vi "Select Searching Method.vi"(8 "error in (no error)":errorcluster) -> (0 "error out":errorcluster, 1 "To Date Field":string, 2 "From Date Field":string, 3 "Selection Type":string)   [LabVIEW 2017]
panel:
  out "Description":string
  in  "Search Type":string(combo)="Date&Time"
  in  "Select":bool
  in  "OK":bool
  # "o selecting this method you can search the"
  # "Select The Searching Method"
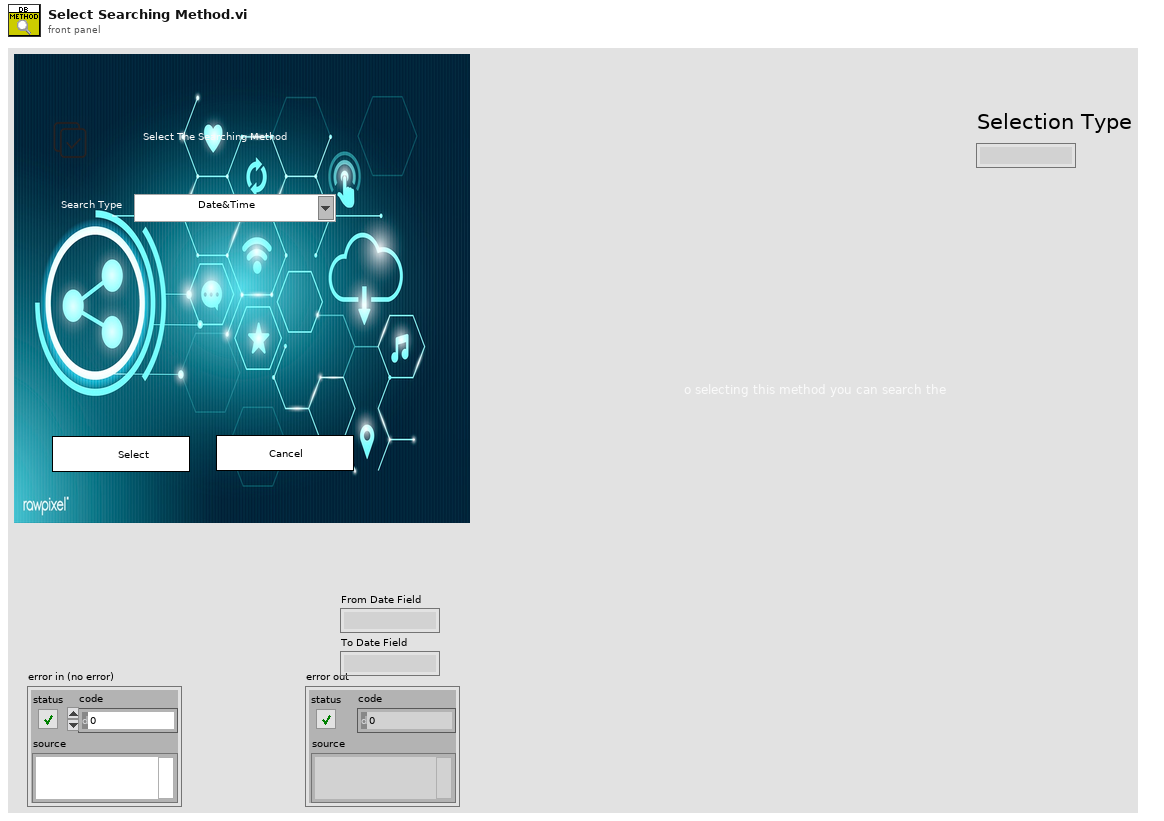
[diagram p1: front panel]
types:
  T1 = cluster{"Search Type":string, "Old Selection Type":string, "Description":string}
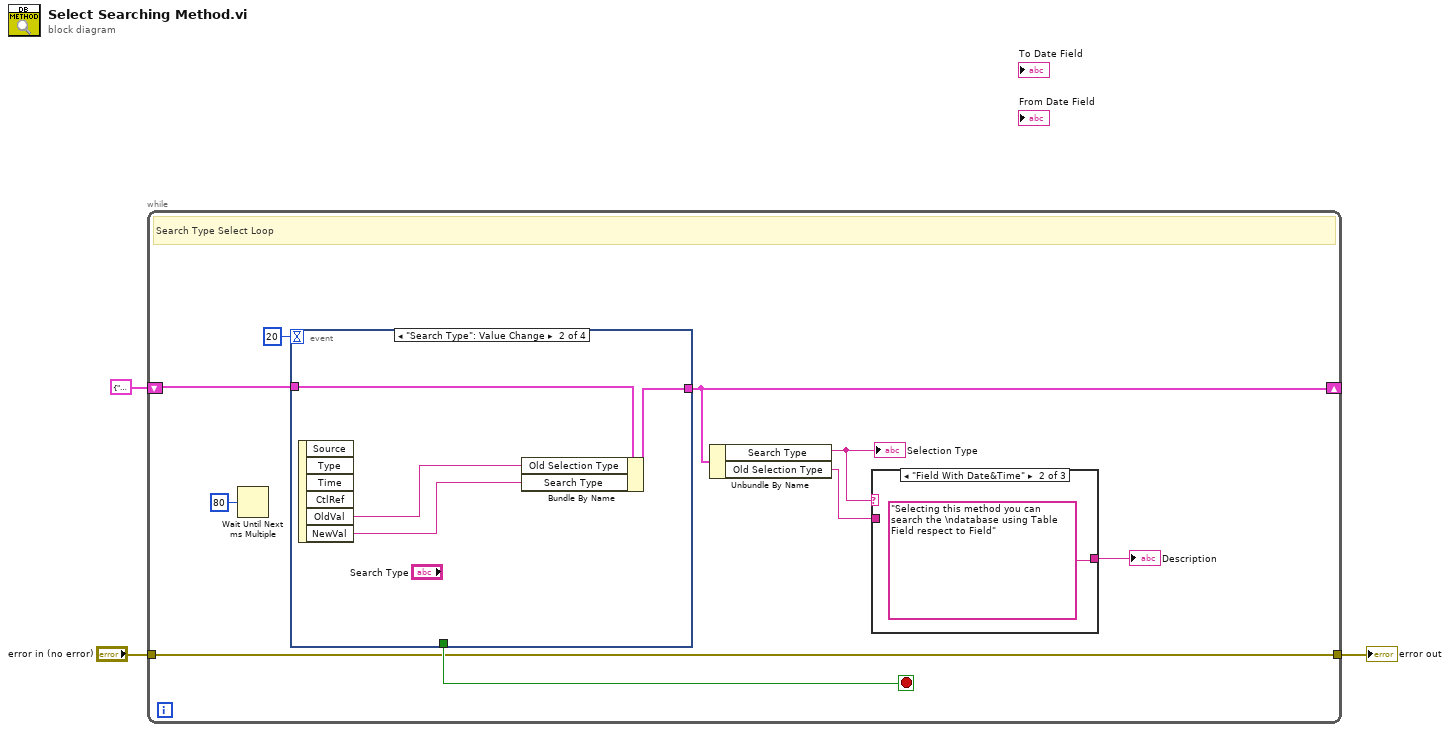
[diagram p0: block diagram]
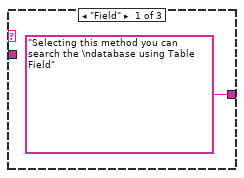
[diagram p2: hidden frame]
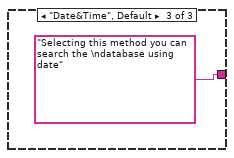
[diagram p3: hidden frame]
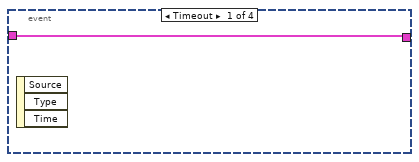
[diagram p4: hidden frame]
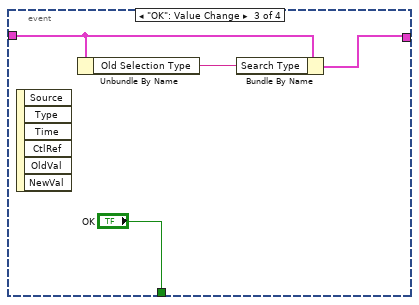
[diagram p5: hidden frame]
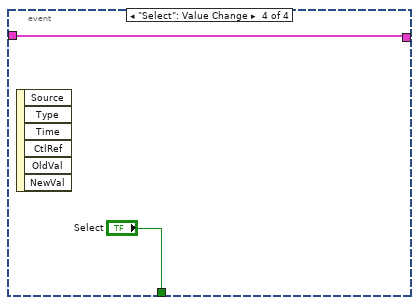
[diagram p6: hidden frame]
diagram:
  n1 = while {
    shift-right: [w9] -> _
    shift-left: T1 {"Search Type"="Date&Time", "Old Selection Type"="", "Description"=""} -> [w10]
    tunnel: [w4] -> w2
    tunnel: "error in (no error)" -> [w4]
    stop <- w8 stop-if-true
    # "Search Type Select Loop"
    n2 = Wait Until Next ms Multiple(millisecond multiple=u32 80) -> ()  [unwired: 1 out]
    n3 = event shown="[1] \"Search Type\": Value Change" {
      selector: _ -> [_ _ _ _]
      dyn-events: _ -> [_ _ _ _]
      timeout: 20 -> [_ _ _ _]
      tunnel: w10 -> [w16 w20 w24 w26]
      tunnel: [w16 w19 w23 w26] -> w9
      tunnel: [_ _ "OK" "Select"] -> w8
      event Timeout {
        n4 = event-data() -> ()  [unwired: 1 in, 3 out]
      }
      event "Search Type": Value Change {
        n5 = event-data() -> ("OldVal"=w18:string, "NewVal"=w17:string)  [unwired: 1 in, 4 out]
        n6 = Bundle By Name(cluster=w20, "Old Selection Type"=w18, "Search Type"=w17) -> (w19:T1)
      }
      event "OK": Value Change {
        n7 = event-data() -> ()  [unwired: 1 in, 6 out]
        n8 = Unbundle By Name(w24) -> ("Old Selection Type"=w22:string)
        n9 = Bundle By Name(cluster=w24, "Search Type"=w22) -> (w23:T1)
      }
      event "Select": Value Change {
        n10 = event-data() -> ()  [unwired: 1 in, 6 out]
      }
    }
    n11 = Unbundle By Name(w9) -> ("Search Type"=w7:string, "Old Selection Type"=w6:string)
    "Selection Type" <- w7
    n12 = case shown="\"Field With Date&Time\"" w7 {
      tunnel: w6 -> [_ _ _]
      tunnel: ["Selecting this method you can search the \ndatabase using Table Field" "Selecting this method you can search the \ndatabase using Table Field respect to Field" "Selecting this method you can search the \ndatabase using date"] -> w5
      frame "Field" {
      }
      frame "Field With Date&Time" {
      }
      frame "Date&Time", Default {
      }
    }
    "Description" <- w5
  }
  "error out" <- w2
